vi "NAfull.vi"() -> ()   [LabVIEW 2012]
uses:
  <vilib>/Utility/miscctls.llb/LVPointDoubleTypeDef.ctl
  <vilib>/Utility/error.llb/DialogType.ctl
panel:
  in  "#Points":dbl(ring)=100.0 items=["10"=10.0, "50"=50.0, "100"=100.0, "200"=200.0, "500"=500.0, "1000"=1000.0]
  in  "Stop":dbl=4000.0 min=34.0 max=4500.0
  in  "Start":dbl=50.0 min=34.0 max=4500.0
  out "ID":string
  in  "RF Power (dB)":dbl(slide)=-31.5 min=-31.5 max=0.0 step=0.5
  in  "Markers":bool=TRUE
  out "Delta":T1
  out "Cursor 2":T1
  out "Cursor 1":T1
  in  "RUN":bool=TRUE
  in  "External\nAtten.":dbl
  in  "Y Scale\nMax":dbl=15.0
  in  "Y Scale\nMin":dbl=-60.0
  in  "Auto\nY Axis":bool
  in  "File\nSave":bool
  in  "Take Cal\nData":bool
  in  "Cal On":bool
  in  "Trace\nHold":bool
  in  "stop":bool
  out "CalData":cluster{dbl[], dbl[]}
  out "Trace":cluster{dbl[], dbl[]}
  out "scope":cluster{dbl[], "trace":dbl[]}[](graph)
  # "(MHz)"
  # "Windfreak"
  # "Technologies, LLC"
  # "Min"
  # "Max"
  # "2013"
  # "Do not unplug USB Cable."
  # "v1.0b"
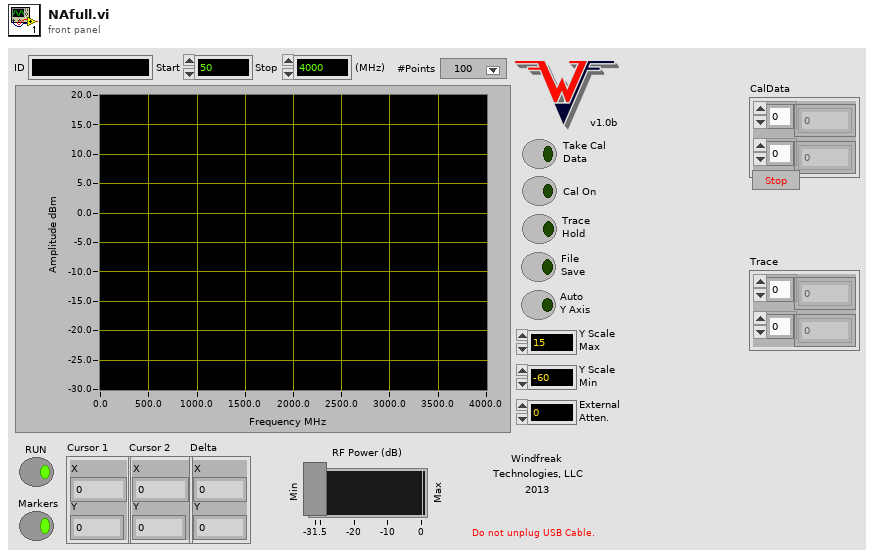
[diagram p1: front panel]
types:
  T1 = typedef "LVPointDoubleTypeDef.ctl" = cluster{"X":dbl, "Y":dbl}
  T2 = enum8{"Enabled", "Disabled", "Disabled and Grayed Out"}
  T3 = typedef "DialogType.ctl" = u16
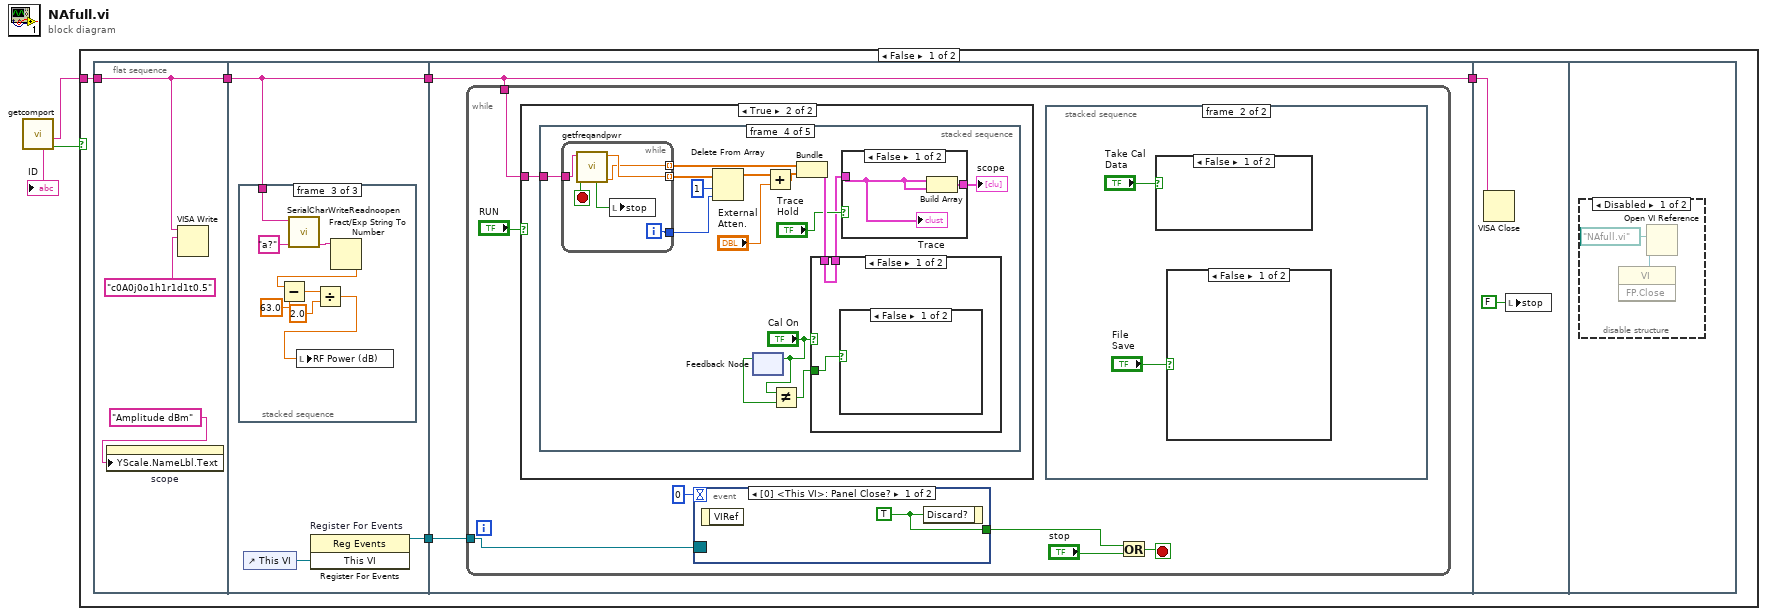
[diagram p0: block diagram]
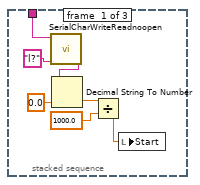
[diagram p2: hidden frame]
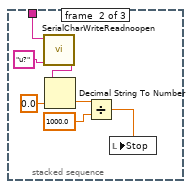
[diagram p3: hidden frame]
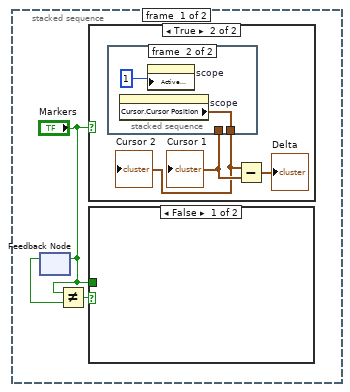
[diagram p4: hidden frame]
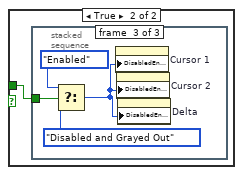
[diagram p5: hidden frame]
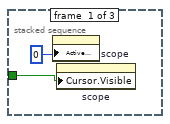
[diagram p6: hidden frame]
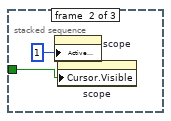
[diagram p7: hidden frame]
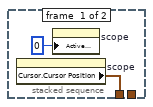
[diagram p9: hidden frame]
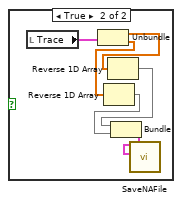
[diagram p10: hidden frame]
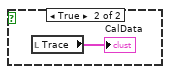
[diagram p11: hidden frame]
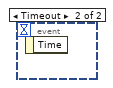
[diagram p12: hidden frame]
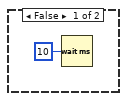
[diagram p13: hidden frame]
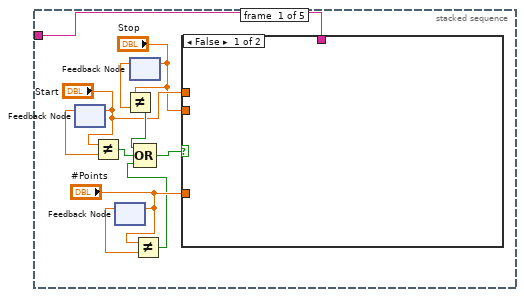
[diagram p14: hidden frame]
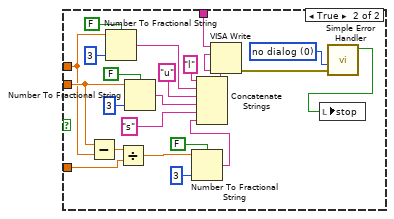
[diagram p15: hidden frame]
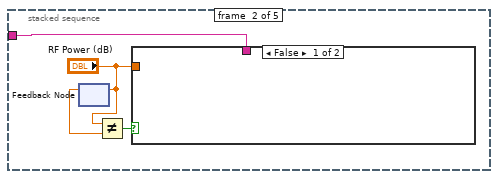
[diagram p16: hidden frame]
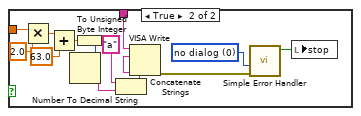
[diagram p17: hidden frame]
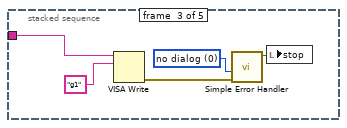
[diagram p18: hidden frame]
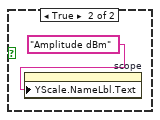
[diagram p19: hidden frame]
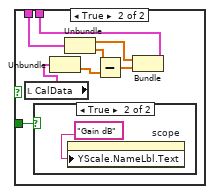
[diagram p20: hidden frame]
diagram:
  n1 = call "getcomport.vi"() -> ("No Devices"=w1:bool, "Port"=w2:string, "Device"=→"ID":string)  [unwired: 9 in]
  n2 = case shown="False" w1 {
    tunnel: w2 -> [w4 _]
    frame False {
      n3 = flat-sequence {
        tunnel: [w9] -> w8
        tunnel: w4 -> [w9]
        tunnel: w8 -> [w14]
        tunnel: [w14] -> w7
        tunnel: [w13] -> w6
        tunnel: w7 -> [w38]
        tunnel: [w38] -> w5
        tunnel: w6 -> [w37]
        tunnel: w5 -> [w187]
        frame #0 {
          n4 = property on="scope" class="XYGraph (strict)"("YScale.NameLbl.Text"="Amplitude dBm" ("Y Scale.Name Label.Text")) -> ()  [unwired: 2 in, 2 out]
          n5 = VISA Write(VISA resource name=w9, write buffer="c0A0j0o1h1r1d1t0.5" ("string")) -> ()  [unwired: 1 in, 3 out]
        }
        frame #1 {
          n6 = stacked-sequence {
            tunnel: w14 -> [w15 w22 w30]
            frame #0 {
              n7 = call "SerialCharWriteReadnoopen.vi"("VISA resource name"=w15, "write buffer"="l?") -> ("read buffer"=w18:string)  [unwired: 8 in]
              n8 = Decimal String To Number(string=w18, default (0L)=0.0 ("default (0 I32)")) -> (number=w20:dbl)  [unwired: 1 in, 1 out]
              n9 = Divide(x=w20, y=1000.0) -> (x/y=w16:dbl)
              n10 = local write "Start"(w16) -> ()
            }
            frame #1 {
              n11 = call "SerialCharWriteReadnoopen.vi"("VISA resource name"=w22, "write buffer"="u?") -> ("read buffer"=w25:string)  [unwired: 8 in]
              n12 = Decimal String To Number(string=w25, default (0L)=0.0 ("default (0 I32)")) -> (number=w27:dbl)  [unwired: 1 in, 1 out]
              n13 = Divide(x=w27, y=1000.0) -> (x/y=w23:dbl)
              n14 = local write "Stop"(w23) -> ()
            }
            frame #2 {
              n15 = call "SerialCharWriteReadnoopen.vi"("VISA resource name"=w30, "write buffer"="a?") -> ("read buffer"=w32:string)  [unwired: 8 in]
              n16 = Fract/Exp String To Number(string=w32) -> (number=w36:dbl)  [unwired: 3 in, 1 out]
              n17 = Subtract(x=w36, y=63.0) -> (x-y=w35:dbl)
              n18 = Divide(x=w35, y=2.0) -> (x/y=w29:dbl)
              n19 = local write "RF Power (dB)"(w29) -> ()
            }
          }
          n20 = control-ref of="This VI"() -> (w12:refnum<vi>)
          n21 = register-events "Register For Events"(w12) -> (reference out=w13:refnum<event-registration>)  [unwired: 2 in, 1 out]
        }
        frame #2 {
          n22 = while {
            tunnel: w38 -> [w44]
            tunnel: w37 -> [w39]
            stop <- w43 stop-if-true
            n23 = case shown="True" "RUN" {
              tunnel: w44 -> [_ w76]
              frame False {
                n24 = Wait (ms)(milliseconds to wait=u32 10) -> ()  [unwired: 1 out]
              }
              frame True {
                n25 = stacked-sequence {
                  tunnel: w76 -> [w82 w110 w131 w144 _]
                  frame #0 {
                    n26 = feedback #1() -> (w87:dbl)  [unwired: 1 in]
                    n27 = feedback-in #1("Start") -> ()
                    n28 = Not Equal?(x="Start", y=w87) -> (x != y?=w86:bool)
                    n29 = feedback #2() -> (w79:dbl)  [unwired: 1 in]
                    n30 = feedback-in #2("#Points") -> ()
                    n31 = feedback #3() -> (w85:dbl)  [unwired: 1 in]
                    n32 = Not Equal?(x="Stop", y=w85) -> (x != y?=w84:bool)
                    n33 = feedback-in #3("Stop") -> ()
                    n34 = Not Equal?(x="#Points", y=w79) -> (x != y?=w77:bool)
                    n35 = Compound Arithmetic op=OR(w84, w86, w77) -> (w83:bool)
                    n36 = case shown="False" w83 {
                      tunnel: w82 -> [_ w107]
                      tunnel: "Start" -> [_ w98]
                      tunnel: "Stop" -> [_ w99]
                      tunnel: "#Points" -> [_ w91]
                      frame False {
                      }
                      frame True {
                        w90 = T3 0 items=["no dialog", "OK message", "continue or stop message", "OK message + warnings", "continue/stop + warnings"] ("type of dialog (OK msg:1)")
                        n37 = Subtract(x=w99, y=w98) -> (x-y=w97:dbl)
                        n38 = Number To Fractional String(use system decimal point (T)=FALSE, number=w98, precision (6)=i16 3) -> (F-format string=w104:string)  [unwired: 1 in]
                        n39 = Divide(x=w97, y=w91) -> (x/y=w93:dbl)
                        n40 = Number To Fractional String(use system decimal point (T)=FALSE, number=w99, precision (6)=i16 3) -> (F-format string=w100:string)  [unwired: 1 in]
                        n41 = Number To Fractional String(use system decimal point (T)=FALSE, number=w93, precision (6)=i16 3) -> (F-format string=w92:string)  [unwired: 1 in]
                        n42 = Concatenate Strings("l" ("string"), w104, "u" ("string"), w100, "s" ("string"), w92) -> (w109:string)
                        n43 = VISA Write(VISA resource name=w107, write buffer=w109) -> (error out=w88:errorcluster)  [unwired: 1 in, 2 out]
                        n44 = call <vilib>:"Simple Error Handler.vi"("type of dialog (OK msg:1)"=w90, "error in (no error)"=w88) -> ("error?"=w89:bool)  [unwired: 7 out]
                        n45 = local write "stop"(w89) -> ()
                      }
                    }
                  }
                  frame #1 {
                    n46 = feedback #4() -> (w111:dbl)  [unwired: 1 in]
                    n47 = feedback-in #4("RF Power (dB)") -> ()
                    n48 = Not Equal?(x="RF Power (dB)", y=w111) -> (x != y?=w113:bool)
                    n49 = case shown="False" w113 {
                      tunnel: "RF Power (dB)" -> [_ w122]
                      tunnel: w110 -> [_ w117]
                      frame False {
                      }
                      frame True {
                        w115 = T3 0 items=["no dialog", "OK message", "continue or stop message", "OK message + warnings", "continue/stop + warnings"] ("type of dialog (OK msg:1)")
                        n50 = Multiply(x=w122, y=2.0) -> (x*y=w124:dbl)
                        n51 = Add(x=w124, y=63.0) -> (x+y=w126:dbl)
                        n52 = To Unsigned Byte Integer(number=w126) -> (unsigned 8bit integer=w119:u8)
                        n53 = Number To Decimal String(number=w119) -> (decimal integer string=w121:string)  [unwired: 1 in]
                        n54 = Concatenate Strings("a" ("element"), w121) -> (w118:string)
                        n55 = VISA Write(VISA resource name=w117, write buffer=w118) -> (error out=w114:errorcluster)  [unwired: 1 in, 2 out]
                        n56 = call <vilib>:"Simple Error Handler.vi"("type of dialog (OK msg:1)"=w115, "error in (no error)"=w114) -> ("error?"=w116:bool)  [unwired: 7 out]
                        n57 = local write "stop"(w116) -> ()
                      }
                    }
                  }
                  frame #2 {
                    w128 = T3 0 items=["no dialog", "OK message", "continue or stop message", "OK message + warnings", "continue/stop + warnings"] ("type of dialog (OK msg:1)")
                    n58 = VISA Write(VISA resource name=w131, write buffer="g1" ("string")) -> (error out=w129:errorcluster)  [unwired: 1 in, 2 out]
                    n59 = call <vilib>:"Simple Error Handler.vi"("type of dialog (OK msg:1)"=w128, "error in (no error)"=w129) -> ("error?"=w127:bool)  [unwired: 7 out]
                    n60 = local write "stop"(w127) -> ()
                  }
                  frame #3 {
                    n61 = while {
                      tunnel: w144 -> [w169]
                      tunnel: [w167] -> w146 mode=indexing
                      tunnel: [w166] -> w141
                      tunnel: [w165] -> w142 mode=indexing
                      i -> [w166]
                      stop <- w168 stop-if-true
                      n62 = call "getfreqandpwr.vi"("VISA resource name"=w169) -> ("Freq"=w165:dbl, "RF Detector Pwr dBm"=w167:dbl, "error?"=w164:bool, "EOS"=w168:bool)  [unwired: 7 in]
                      n63 = local write "stop"(w164) -> ()
                    }
                    n64 = Delete From Array(array=w146, length=1, index=w141) -> (array with subset deleted=w137:dbl[])  [unwired: 1 out]
                    n65 = feedback #5() -> (w135:bool)  [unwired: 1 in]
                    n66 = feedback-in #5("Cal On") -> ()
                    n67 = Add(x=w137, y="External\nAtten.") -> (x+y=w138:dbl[])
                    n68 = Not Equal?(x="Cal On", y=w135) -> (x != y?=w133:bool)
                    n69 = Bundle(w142, w138) -> (w139:cluster{dbl[], dbl[]})  [unwired: 1 in]
                    n70 = case shown="False" "Cal On" {
                      tunnel: w139 -> [w148 w157]
                      tunnel: [w148 w152] -> w132
                      tunnel: w133 -> [w147 w150]
                      frame False {
                        n71 = case shown="False" w147 {
                          frame False {
                          }
                          frame True {
                            n72 = property on="scope" class="XYGraph (strict)"("YScale.NameLbl.Text"="Amplitude dBm" ("Y Scale.Name Label.Text")) -> ()  [unwired: 2 in, 2 out]
                          }
                        }
                      }
                      frame True {
                        n73 = local read "CalData"() -> (w151:cluster{dbl[], dbl[]})
                        n74 = case shown="True" w150 {
                          frame False {
                          }
                          frame True {
                            n75 = property on="scope" class="XYGraph (strict)"("YScale.NameLbl.Text"="Gain dB" ("Y Scale.Name Label.Text")) -> ()  [unwired: 2 in, 2 out]
                          }
                        }
                        n76 = Unbundle(w151) -> (w156:dbl[])  [unwired: 1 out]
                        n77 = Unbundle(w157) -> (w153:dbl[], w155:dbl[])
                        n78 = Subtract(x=w155, y=w156) -> (x-y=w154:dbl[])
                        n79 = Bundle(w153, w154) -> (w152:cluster{dbl[], dbl[]})  [unwired: 1 in]
                      }
                    }
                    n80 = case shown="False" "Trace\nHold" {
                      tunnel: [w160 w163] -> w143
                      tunnel: w132 -> [w159 w162]
                      frame False {
                        n81 = Build Array(w159, w159) -> (w160:cluster{dbl[], dbl[]}[])
                        "Trace" <- w159
                      }
                      frame True {
                        n82 = local read "Trace"() -> (w161:cluster{dbl[], dbl[]})
                        n83 = Build Array(w162, w161) -> (w163:cluster{dbl[], dbl[]}[])
                      }
                    }
                    "scope" <- w143
                  }
                  frame #4 {
                    n84 = feedback #6() -> (w170:bool)  [unwired: 1 in]
                    n85 = feedback-in #6("Auto\nY Axis") -> ()
                    n86 = feedback #7() -> (w172:dbl)  [unwired: 1 in]
                    n87 = feedback-in #7("Y Scale\nMax") -> ()
                    n88 = feedback #8() -> (w173:dbl)  [unwired: 1 in]
                    n89 = feedback-in #8("Y Scale\nMin") -> ()
                    n90 = Not Equal?(x="Auto\nY Axis", y=w170) -> (x != y?=w178:bool)
                    n91 = Not Equal?(x="Y Scale\nMax", y=w172) -> (x != y?=w176:bool)
                    n92 = Not Equal?(x="Y Scale\nMin", y=w173) -> (x != y?=w177:bool)
                    n93 = Compound Arithmetic op=OR(w178, w176, w177) -> (w175:bool)
                    n94 = case shown="True" w175 {
                      tunnel: "Auto\nY Axis" -> [_ w182]
                      tunnel: "Y Scale\nMax" -> [_ w181]
                      tunnel: "Y Scale\nMin" -> [_ w180]
                      frame False {
                      }
                      frame True {
                        n95 = case shown="False" w182 {
                          tunnel: w181 -> [w184 _]
                          tunnel: w180 -> [w183 _]
                          frame False {
                            n96 = property on="scope" class="XYGraph (strict)"("YScale.Maximum"=w184, "YScale.Minimum"=w183) -> ()  [unwired: 2 in, 2 out]
                          }
                          frame True {
                            n97 = property on="scope" class="XYGraph (strict)"("YScale.ScaleFit"=u8 1 ("Y Scale.Scale Fit")) -> ()  [unwired: 2 in, 2 out]
                          }
                        }
                      }
                    }
                  }
                }
              }
            }
            n98 = event shown="[0] <This VI>: Panel Close?" {
              selector: w39 -> [_ _]
              dyn-events: _ -> [_ _]
              timeout: 0 -> [_ _]
              tunnel: [w74 _] -> w41
              event Panel Close? {
                w74 = TRUE ("Discard?")
                n99 = event-data() -> ()  [unwired: 1 in, 1 out]
                n100 = event-data("Discard?"=w74) -> ()  [unwired: 1 in, 1 out]
              }
              event Timeout {
                n101 = event-data() -> ()  [unwired: 1 in, 1 out]
              }
            }
            n102 = stacked-sequence {
              frame #0 {
                n103 = feedback #9() -> (w48:bool)  [unwired: 1 in]
                n104 = feedback-in #9("Markers") -> ()
                n105 = Not Equal?(x="Markers", y=w48) -> (x != y?=w47:bool)
                n106 = case shown="True" "Markers" {
                  frame False {
                  }
                  frame True {
                    n107 = stacked-sequence {
                      tunnel: [w61 _] -> w59
                      tunnel: [_ w63] -> w58
                      frame #0 {
                        n108 = property on="scope" class="XYGraph (strict)"() -> ("Cursor.Cursor Position"=w61:T1)  [unwired: 2 in, 2 out]
                        n109 = property on="scope" class="XYGraph (strict)"("Active Cursor"=u32 0) -> ()  [unwired: 2 in, 2 out]
                      }
                      frame #1 {
                        n110 = property on="scope" class="XYGraph (strict)"() -> ("Cursor.Cursor Position"=w63:T1)  [unwired: 2 in, 2 out]
                        n111 = property on="scope" class="XYGraph (strict)"("Active Cursor"=u32 1) -> ()  [unwired: 2 in, 2 out]
                      }
                    }
                    "Cursor 1" <- w59
                    "Cursor 2" <- w58
                    n112 = Subtract(x=w58, y=w59) -> (x-y=→"Delta":T1)
                  }
                }
                n113 = case shown="False" w47 {
                  tunnel: "Markers" -> [_ w49]
                  frame False {
                  }
                  frame True {
                    n114 = stacked-sequence {
                      tunnel: w49 -> [w51 w52 w57]
                      frame #0 {
                        n115 = property on="scope" class="XYGraph (strict)"("Active Cursor"=u32 0) -> ()  [unwired: 2 in, 2 out]
                        n116 = property on="scope" class="XYGraph (strict)"("Cursor.Visible"=w51) -> ()  [unwired: 2 in, 2 out]
                      }
                      frame #1 {
                        n117 = property on="scope" class="XYGraph (strict)"("Active Cursor"=u32 1) -> ()  [unwired: 2 in, 2 out]
                        n118 = property on="scope" class="XYGraph (strict)"("Cursor.Visible"=w52) -> ()  [unwired: 2 in, 2 out]
                      }
                      frame #2 {
                        n119 = Select(t=T2."Enabled" ("Disabled"), s=w57, f=T2."Disabled and Grayed Out" ("Disabled")) -> (s? t:f=w54:T2)
                        n120 = property on="Cursor 1" class="Clust (strict)"("DisabledEnum"=w54) -> ()  [unwired: 2 in, 2 out]
                        n121 = property on="Cursor 2" class="Clust (strict)"("DisabledEnum"=w54) -> ()  [unwired: 2 in, 2 out]
                        n122 = property on="Delta" class="Clust (strict)"("DisabledEnum"=w54) -> ()  [unwired: 2 in, 2 out]
                      }
                    }
                  }
                }
              }
              frame #1 {
                n123 = case shown="False" "Take Cal\nData" {
                  frame False {
                  }
                  frame True {
                    n124 = local read "Trace"() -> (→"CalData":cluster{dbl[], dbl[]})
                  }
                }
                n125 = case shown="False" "File\nSave" {
                  frame False {
                  }
                  frame True {
                    n126 = local read "Trace"() -> (w67:cluster{dbl[], dbl[]})
                    n127 = Unbundle(w67) -> (w72:dbl[], w71:dbl[])
                    n128 = Reverse 1D Array(array=w71) -> (reversed array=w69:dbl[])
                    n129 = Reverse 1D Array(array=w72) -> (reversed array=w70:dbl[])
                    n130 = Bundle(w70, w69) -> (w68:cluster{dbl[], dbl[]})  [unwired: 1 in]
                    n131 = call "SaveNAFile.vi"("XY"=w68) -> ()  [unwired: 7 in, 1 out]
                  }
                }
              }
            }
            n132 = Or(x=w41, y="stop") -> (x .or. y?=w43:bool)
          }
        }
        frame #3 {
          n133 = VISA Close(VISA resource name=w187) -> ()  [unwired: 1 in, 1 out]
          n134 = local write "stop"(FALSE ("stop")) -> ()
        }
        frame #4 {
          n135 = disable-structure shown="Disabled" {
            frame Disabled {
              n136 = Open VI Reference(vi path=path "NAfull.vi") -> (vi reference=w188:refnum<vi>)  [unwired: 5 in, 1 out]
              n137 = invoke class="VI" method="FP.Close"(reference=w188) -> ()  [unwired: 2 in, 3 out]
            }
            frame Enabled {
            }
          }
        }
      }
    }
    frame True {
      n138 = Open VI Reference(vi path=path "NAfull.vi") -> (vi reference=w190:refnum<vi>)  [unwired: 5 in, 1 out]
      n139 = invoke class="VI" method="FP.Close"(reference=w190) -> ()  [unwired: 2 in, 3 out]
    }
  }
